vi "Verify Minor Frame Command.vi"(5 "Instruction ID":i32, 6 "Pointers":T1={"Major Command Pointer"=2206, "Major Data Pointer"=2206, "Minor Command Pointer"=2206, "Minor Data Pointer"=2206}, 7 "Target IC (1-8)":u8, 8 "error in (no error)":errorcluster, 11 "BC Major Frame in":refnum<class "BC Major Frame.lvclass">) -> (0 "error out":errorcluster, 3 "BC Major Frame out":refnum<class "BC Major Frame.lvclass">, 4 "Pointers out":T1={"Major Command Pointer"=0, "Major Data Pointer"=0, "Minor Command Pointer"=2206, "Minor Data Pointer"=2206})   [LabVIEW 2016, in "BC Major Frame.lvclass"]
uses:
  BC Major Frame.lvclass
  Data Pointers.ctl
  Frames & Messages/TypeDefs/BC Op Codes - Verbose.ctl
  Frames & Messages/TypeDefs/BC Condition Codes.ctl
  PPLs/FPGA Interface.lvlibp/FPGA Interface/FPGA Interface.lvclass
  BCI-1553 API.lvlib
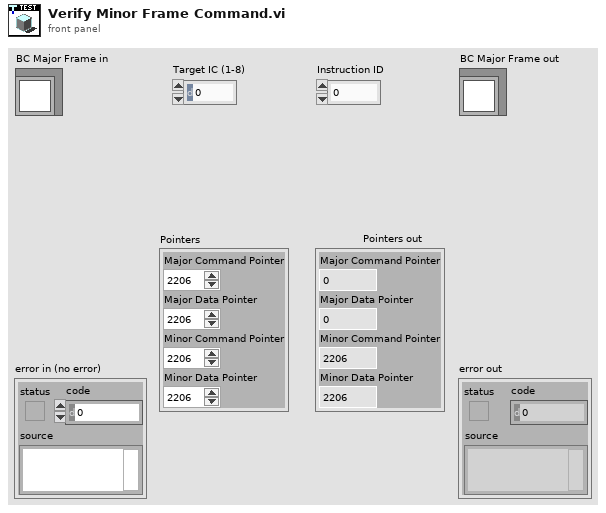
[diagram p1: front panel]
types:
  T1 = typedef "Data Pointers.ctl" = cluster{"Major Command Pointer":u16, "Major Data Pointer":u16, "Minor Command Pointer":u16, "Minor Data Pointer":u16}
  T2 = typedef "BCI-1553 API.lvlib/BC Condition Codes.ctl" = enum16{"GP0 == 1 || LT", "GP1 == 1 || NE", "GP2 == 1", "GP3 == 1", "GP4 == 1", "GP5 == 1", "GP6 == 1", "GP7 == 1", "NORESP", "FMTERR", "GOODBLOCK", "MSKSTATSET", "BADMSG", "1RETRY", "2RETRY", "ALWAYS"}
  T3 = typedef "BCI-1553 API.lvlib/BC Op Codes - Verbose.ctl" = enum16{"EXECUTE MSG", "EXECUTE MSG GO", "JUMP", "CALL SUBROUTINE", "RETURN", "INTERRUPT REQUEST", "HALT", "DELAY", "WAIT FRAME TIMER = 0", "COMPARE FRAME TIMER", "COMPARE MSG TIMER", "LOAD TIME TAG CTR", "LOAD TIME TAG CTR HI", "LOAD FRAME TIMER", "START FRAME TIMER", "PUSH TIME TAG COUNT", "PUSH TIME TAG COUNT HI", "PUSH TIME TAG COUNT BOTH", "PUSH BLOCK STATUS WORD", "PUSH CURRENT VALUE", "PUSH INDIRECT", "WAIT EXT TRIGGER", "EXECUTE AND FLIP", "EXECUTE, FLIP, GO", "WRITE VALUE TO WMI", "WRITE VALUE TO MEM", "DECREMENT RAM, SKIP", "FLAG"}
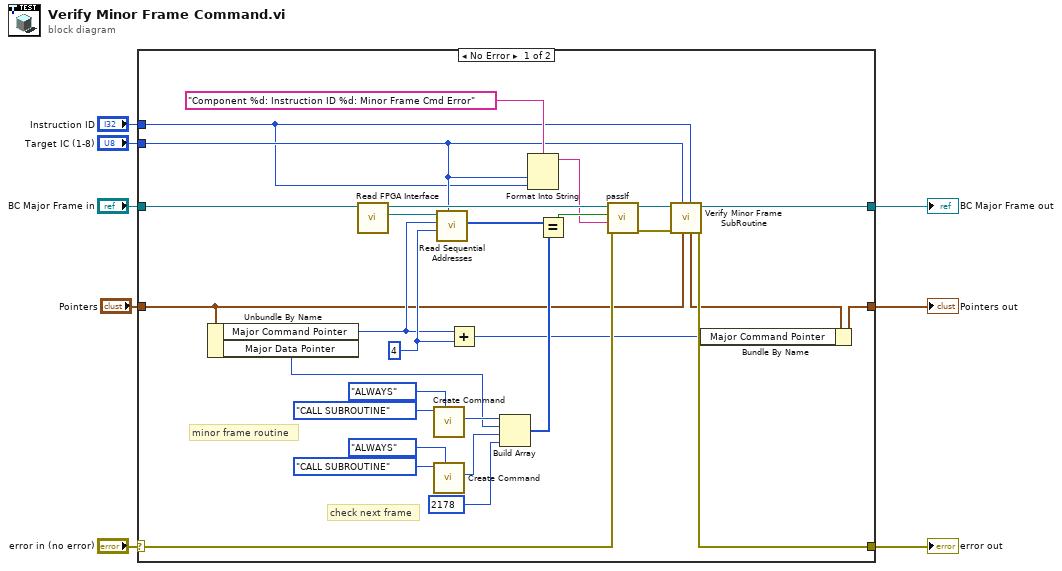
[diagram p0: block diagram]
diagram:
  n1 = case shown="No Error" "error in (no error)" {
    selector: "error in (no error)" -> [w33 w39]
    tunnel: [w15 w39] -> w7
    tunnel: [w16 w38] -> w5
    tunnel: "BC Major Frame in" -> [w37 w38]
    tunnel: "Target IC (1-8)" -> [w18 _]
    tunnel: "Instruction ID" -> [w17 _]
    tunnel: "Pointers" -> [w10 _]
    tunnel: [w11 _] -> w1
    frame No Error {
      w35 = u16 4 ("Addresses to Read")
      # "minor frame routine"
      # "check next frame"
      n2 = Unbundle By Name(w10) -> ("Major Command Pointer"=w14:u16, "Major Data Pointer"=w13:u16)
      n3 = call-dynamic "Read FPGA Interface.vi"("1553 Test in"=w37) -> ("FPGA Interface"=w36:refnum<class "FPGA Interface.lvclass">, "1553 Test out"=w34:refnum<class "BC Major Frame.lvclass">)  [unwired: 8 in, 1 out]
      n4 = call "Create Command.vi"("Condition"=BC_Condition_Codes."ALWAYS", "Op Code"=BC_Op_Codes_-_Verbose."CALL SUBROUTINE") -> ("Instruction"=w28:u16)  [unwired: 8 in, 1 out]
      n5 = call "Create Command.vi"("Condition"=BC_Condition_Codes."ALWAYS", "Op Code"=BC_Op_Codes_-_Verbose."CALL SUBROUTINE") -> ("Instruction"=w27:u16)  [unwired: 8 in, 1 out]
      n6 = call-dynamic "Read Sequential Addresses.vi"("Target IC (1-8)"=w18, "Addresses to Read"=w35, "Starting Address"=w14, "FPGA Interface in"=w36) -> ("Data"=w24:u16[])  [unwired: 6 in, 1 out]
      n7 = Add(x=w14, y=w35) -> (x+y=w12:u16)
      n8 = Build Array(w28, w13, w27, u16 2178) -> (w25:u16[])
      n9 = Format Into String(format string="Component %d: Instruction ID %d: Minor Frame Cmd Error" ("message (\"\")"), w18, w17) -> (resulting string=w19:string)  [unwired: 2 in, 1 out]
      n10 = Equal?(x=w24, y=w25) -> (x = y?=w23:bool)
      n11 = call-dynamic "passIf.vi"("error in (no error)"=w33, "message (\"\")"=w19, "pass"=w23, "TestCase in"=w34) -> ("error out"=w21:errorcluster, "TestCase out"=w22:refnum<class "BC Major Frame.lvclass">)  [unwired: 6 in]
      n12 = call "Verify Minor Frame SubRoutine.vi"("Instruction ID"=w17, "Pointers"=w10, "Target IC (1-8)"=w18, "error in (no error)"=w21, "BC Major Frame in"=w22) -> ("error out"=w15:errorcluster, "BC Major Frame out"=w16:refnum<class "BC Major Frame.lvclass">, "Pointers out"=w9:T1)  [unwired: 4 in]
      n13 = Bundle By Name(cluster=w9, "Major Command Pointer"=w12) -> (w11:T1)
    }
    frame Error {
    }
  }
  "error out" <- w7
  "BC Major Frame out" <- w5
  "Pointers out" <- w1
